vi "Henonbifr.vi"() -> ()   [LabVIEW 2012]
panel:
  out "Bifurcation Diagram of Henon Map":cluster{dbl[], "X's":dbl[]}(graph)
  in  "B":dbl=0.3 format="%.2f"
  out "Progress slider":sgl(slide)=0.99333334 scale=0.0..1.0 scale format="%.2f"
  in  "# of A-samples":i32=150
  in  "Number of Iterates to throw away":i16=100 step=50
  in  "A Stop":dbl=1.4 step=0.01 format="%.4f"
  in  "A Start":dbl step=0.01 format="%.4f"
  in  "Number of Iterates per value of R":i16=150 step=50
  # "2"
  # "{"
  # "Xn+1 = Yn +1-AXn"
  # "The Henon Map:"
  # "Yn+1 = BXn"
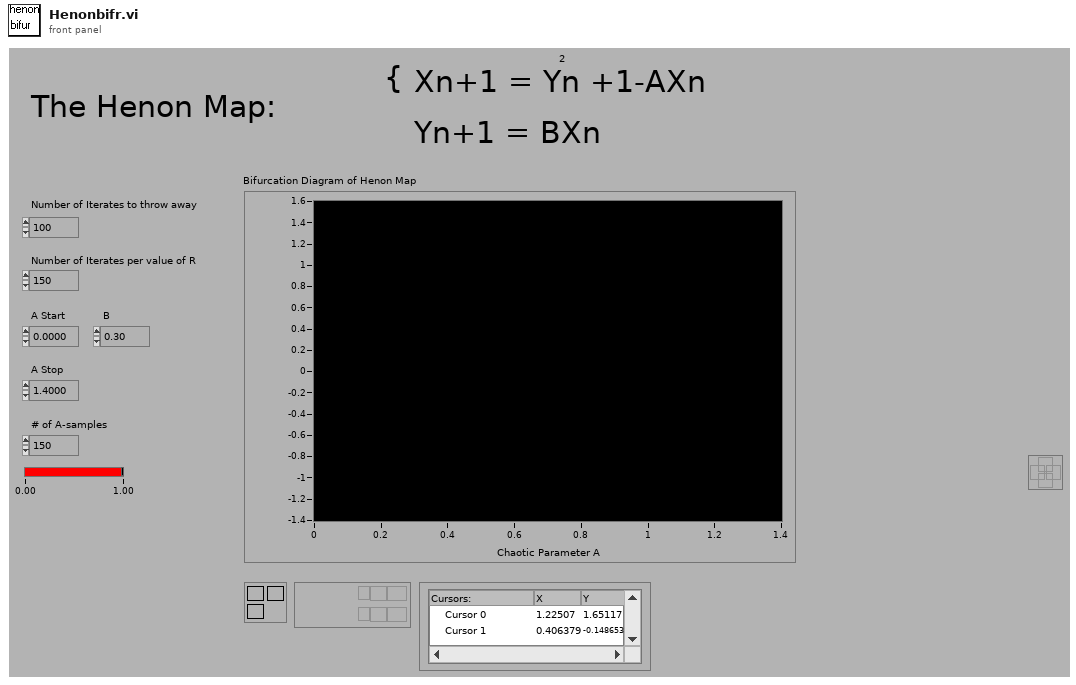
[diagram p1: front panel]
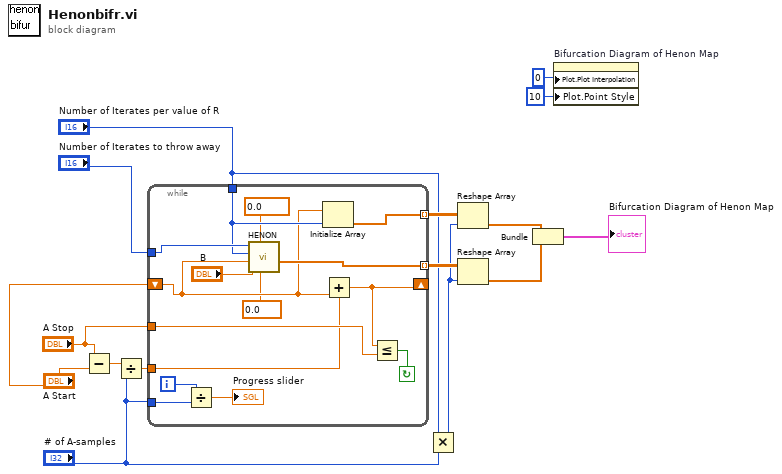
[diagram p0: block diagram]
diagram:
  n1 = Subtract(x="A Stop", y="A Start") -> (x-y=w13:dbl)
  n2 = Divide(x=w13, y="# of A-samples") -> (x/y=w12:dbl)
  n3 = while {
    tunnel: "# of A-samples" -> [w23]
    tunnel: [w25] -> w11 mode=indexing
    tunnel: [w26] -> w9 mode=indexing
    tunnel: w12 -> [w27]
    tunnel: "A Stop" -> [w28]
    tunnel: "Number of Iterates to throw away" -> [w21]
    tunnel: "Number of Iterates per value of R" -> [w20]
    shift-left: "A Start" -> [w19]
    shift-right: [w30] -> _
    i -> [w24]
    stop <- w29 continue-if-true
    n4 = Divide(x=w24, y=w23) -> (x/y=→"Progress slider":dbl)
    n5 = call "HENON.VI"("IV:y"=0.0, "IV: x"=0.0, "B"="B", "A"=w19, "Number of Iterates to compute"=w20, "Number of pre-iterates"=w21) -> ("X's"=w26:dbl[])  [unwired: 3 out]
    n6 = Initialize Array(w19, w20) -> (w25:dbl[])
    n7 = Add(x=w19, y=w27) -> (x+y=w30:dbl)
    n8 = Less Or Equal?(x=w30, y=w28) -> (x <= y?=w29:bool)
  }
  n9 = Multiply(x="Number of Iterates per value of R", y="# of A-samples") -> (x*y=w7:i32)
  n10 = Reshape Array(w11, w7) -> (w10:dbl[])
  n11 = Reshape Array(w9, w7) -> (w8:dbl[])
  n12 = Bundle(w10, "X's"=w8) -> (→"Bifurcation Diagram of Henon Map":cluster{dbl[], "X's":dbl[]})  [unwired: 1 in]
  n13 = property on="Bifurcation Diagram of Henon Map" class="XYGraph (strict)"("Plot.Plot Interpolation"=u8 0, "Plot.Point Style"=u8 10) -> ()  [unwired: 2 in, 2 out]
